vi "Robot Global Data.vi"() -> ()   [LabVIEW 2014]
doc: "This global VI can contain as many global variables as you need. Place a control on the panel, give it a good name. To read or write to it from a VI, drag the icon to the diagram of that VI. You can also drag from the project. Click on the node to change which global you access. You shouldn't have multiple locations writing to a global or it will cause a race-condition."
uses:
  <vilib>/Rock Robotics/WPI/Camera/WPI_CameraImageSize.ctl
  <vilib>/Rock Robotics/WPI/DriverStation/WPI_DriverStationRobotMode2.ctl
panel:
  in  "Manul drive offset Winch 2":dbl
  in  "Manual scale Winch2":dbl
  in  "Lower limit Winch 2":dbl
  in  "upper limit Winch 2":dbl
  in  "Step Inches Winch 2":dbl
  in  "Encoder 2 scale":dbl
  in  "Gripper Open":bool
  in  "Lift Global":bool
  in  "Lower Global":bool
  in  "Sonar Offset":dbl
  in  "Sonar Limit":dbl
  in  "Value 10":dbl
  in  "Value 9":dbl
  in  "Manul drive offset Winch 1":dbl
  in  "Manual scale Winch 1":dbl
  in  "Lower limit Winch 1":dbl
  in  "upper limit Winch 1":dbl
  in  "Step Inches Winch 1":dbl
  in  "Encoder 1 scale":dbl
  in  "Robot Mode":T1
  in  "image size":T2=enum."320x240"
  in  "Enable Vision":bool
  # "INI Values"
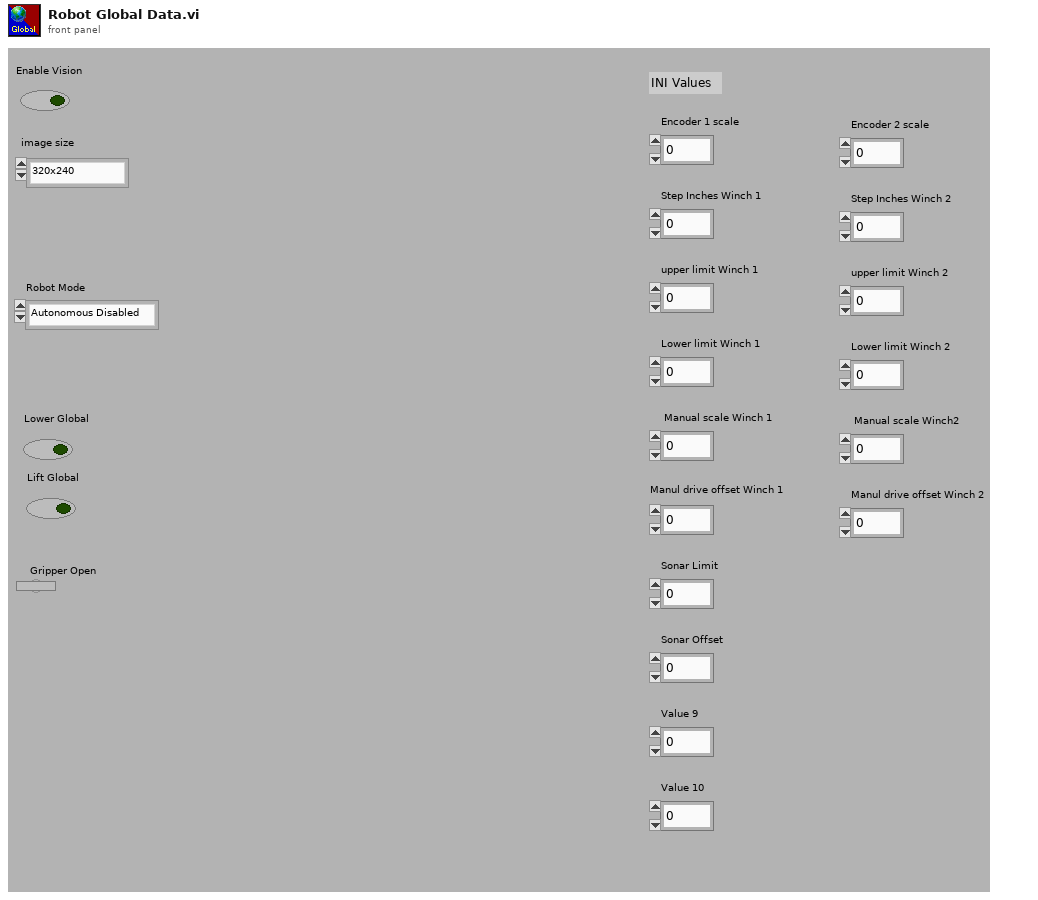
[diagram p1: front panel]
types:
  T1 = typedef "WPI_DriverStationRobotMode2.ctl" = enum16{"Autonomous Disabled", "Autonomous Enabled", "Teleop Disabled", "Teleop Enabled", "Disconnected", "Finish", "Test Disabled", "Test Enabled", "Emergency Stopped"}
  T2 = typedef "WPI_CameraImageSize.ctl" = enum16{"640x480", "320x240", "160x120", "Custom"}
diagram:
